vi "LogWriteToGlobal.vi"(11 "in string":string) -> ()   [LabVIEW 2019]
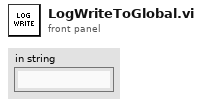
[diagram p1: front panel]
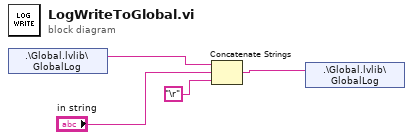
[diagram p0: block diagram]
diagram:
  n1 = shared-variable ".\\Global.lvlib\\GlobalLog"() -> (w4:string)  [unwired: 1 in, 1 out]
  n2 = Concatenate Strings(w4, "in string", "\r") -> (w1:string)
  n3 = shared-variable ".\\Global.lvlib\\GlobalLog"(w1) -> ()  [unwired: 1 in, 1 out]
